vi "Set BandLimits.vi"(6 "parseError? T:Yes":bool=TRUE, 8 "error in (no error)":errorcluster, 9 "Lower Bandlimit (200K)":dbl=200.0 min=1.0 max=200.0, 10 "Upper Bandlimit (200K)":dbl=200.0 min=1.0 max=200.0, 11 "VISA resource name":refnum<visa-resource-name>) -> (0 "error out":errorcluster, 3 "VISA resource name out":refnum<visa-resource-name>)   [LabVIEW 2015, in "JULABO DeviceDriver.lvlib"]
doc: "This VI adjusts the maximum allowed difference between internal and external temperature during heating up and cooling down.\nAdjustable range: <B>0 ... 200 K</B>\n\nNote:\nThis function is not available for instruments which do not support different values for upper and lower bandlimit. Please use <B>JULABO_Configure_SetBand.vi</B> in case your instrument supports only one bandlimit. See operating manual to check whether your instrument supports different values for lower and upper bandlimit.\n\nThis function is not available for devices which do not have an external sensor plug. For these instruments the VI will return an error (-08 INVALID COMMAND)."
uses:
  JULABO DeviceDriver.lvlib
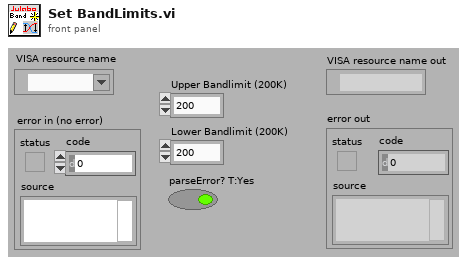
[diagram p1: front panel]
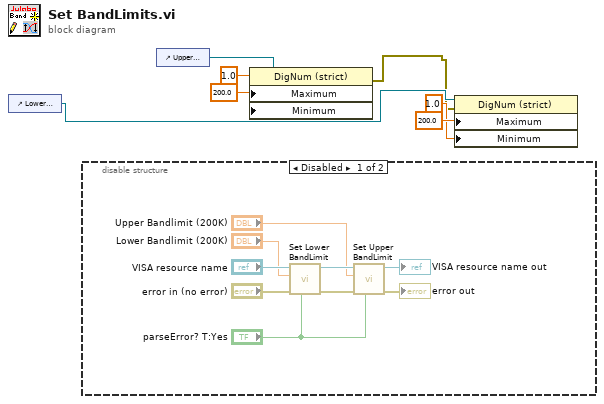
[diagram p0: block diagram]
diagram:
  n1 = control-ref of="Lower Bandlimit (200K)"() -> (w2:refnum<vi>)
  n2 = disable-structure shown="Disabled" {
    frame Disabled {
      n3 = call "Set Lower BandLimit.vi"("parseError? T:Yes"="parseError? T:Yes", "error in (no error)"="error in (no error)", "Lower Bandlimit (200K)"="Lower Bandlimit (200K)", "VISA resource name"="VISA resource name") -> ("error out"=w13:errorcluster, "VISA resource name out"=w14:refnum<visa-resource-name>)  [unwired: 6 in]
      n4 = call "Set Upper BandLimit.vi"("parseError? T:Yes"="parseError? T:Yes", "error in (no error)"=w13, "Upper Bandlimit (200K)"="Upper Bandlimit (200K)", "VISA resource name"=w14) -> ("error out"=→"error out":errorcluster, "VISA resource name out"=→"VISA resource name out":refnum<visa-resource-name>)  [unwired: 6 in]
    }
    frame Enabled {
    }
  }
  n5 = control-ref of="Upper Bandlimit (200K)"() -> (w7:refnum<vi>)
  n6 = property class="DigNum (strict)"(reference=w7, "Maximum"=200.0 ("Wertebereich:Maximum"), "Minimum"=1.0 ("Wertebereich:Minimum")) -> (error out=w1:errorcluster)  [unwired: 1 in, 1 out]
  n7 = property class="DigNum (strict)"(reference=w2, error in=w1, "Maximum"=200.0 ("Wertebereich:Maximum"), "Minimum"=1.0 ("Wertebereich:Minimum")) -> ()  [unwired: 2 out]
